vi "Variant to JSON.vi"(7 "Treatment of Infinity/NaN":T1, 8 "error in (no error)":errorcluster, 10 "Variant":variant) -> (0 "error out":errorcluster, 3 "JSON Value out":refnum<class "JSON Value.lvclass">)   [LabVIEW 2020, in "Library Commun.lvlib" / "Variant JSON.lvlib"]
doc: "Converts a LabVIEW datatype (<b>Variant</b>) into a JSON value. Clusters are converted to JSON Objects. Variants, if empty (void), are converted to null, unless they have attributes, in which case these are converted into a JSON object. \n\nTreatment of Infinity, -Infinity, and Not-a-Number values of floating-point numerics:\n<b>-- Default JSON:</b> write all as nulls.\n<b>-- Extended:</b> use JSON strings for Infinities (\"Infinity\", \"-Infinity\"); NaN still null.\n<b>-- LabVIEW extentions</b> (compatable with the LabVIEW JSON primatives): Infinity, -Infinity, NaN (not in quotes)\n\nNote that the LabVIEW extentions are not valid JSON. The Extended option <b>is</b> valid JSON, but not all JSON parsers will process strings as numeric values.\n\nMore information on http://lavag.org/topic/16217-cr-json-labview"
uses:
  Variant JSON.lvlib
  JSON Value/JSON Value.lvclass
  JSON Scalar/Infinity&NaN.ctl
  <vilib>/Utility/VariantDataType/Type.ctl
  JSON Object/JSON Object.lvclass
  C:/Users/ngarcin/OneDrive - Altyor/Standard TB/Class/JSON API/JSON Value/JSON Value.lvclass
  JSON Array/JSON Array.lvclass
  JSON Array/JSON Array.lvclass/JSON Array.ctl
  JSON Value/Set from JSON string.vi
  JSON Scalar/JSON Scalar.lvclass
  JSON Scalar/Set Null.vi
  JSON Scalar/Set I32.vi
  JSON Scalar/Set I64.vi
  JSON Scalar/Set U32.vi
  JSON Scalar/Set U64.vi
  JSON Scalar/Set SGL.vi
  JSON Scalar/Set EXT.vi
  JSON Scalar/Set Boolean.vi
  JSON Scalar/Set Path.vi
  JSON Scalar/Set Timestamp.vi
  Get Polymorphic/JSON GetSet.lvlib
  <vilib>/Utility/VariantDataType/VariantType.lvlib
  <userlib>/_OpenG.lib/lvdata/lvdata.llb/openg_variant.lvlib
  support/JSON support.lvlib
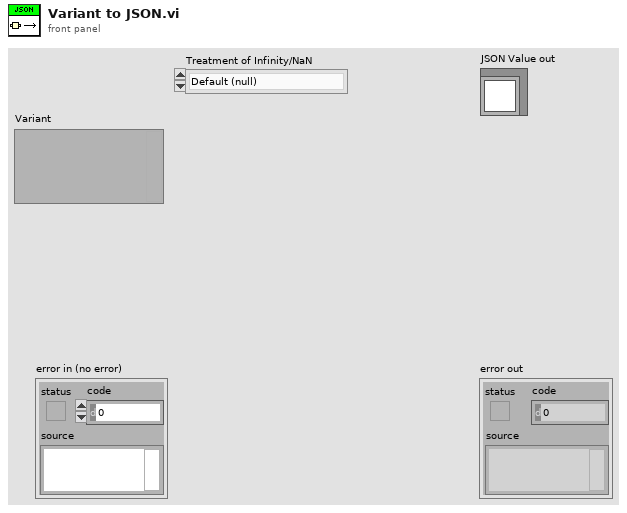
[diagram p1: front panel]
types:
  T1 = typedef "Library Commun.lvlib/JSON support.lvlib/Infinity&NaN.ctl" = enum16{"Default (null)", "Extended", "LabVIEW extensions"}
  T2 = typedef "VariantType.lvlib/Type.ctl" = enum8{"Invalid Type", "Void", "I8", "I16", "I32", "I64", "U8", "U16", "U32", "U64", "Single Float", "Double Float", "Extended Float", "Single Complex", "Double Complex", "Extended Complex", "Enum U8", "Enum U16", "Enum U32", "Enum U64", "Single Float With Unit", "Double Float With Unit", "Extended Float With Unit", "Single Complex with Unit", "Double Complex with Unit", "Extended Complex with Unit", "Boolean", "String", "Path", "Picture", "Tag", "Array", "Cluster", "Variant", "LV Variant", "Waveform", "Timestamp", "Digital Waveform", "Digital Data", "ExpressData", "Refnum", "External Data", "VI", "Poly VI", "LabVIEW Class Instance", "Fixed Point"}
  T3 = typedef "VariantType.lvlib/RefnumType.ctl" = enum16{"NotARefnum", "UnknownRefnum", "Generic", "Datalog", "ByteStream", "Device", "Occurence", "TCPNetConnection", "Auto", "Menu", "Imaq", "Hardware", "DataSocket", "Visa", "IVI", "UDPNetConnection", "Notifier", "Queue", "Irda", "EventReg", "DotNet", "UserEvent", "Callback", "UNUSED_EMPTY_POSITION", "BlueToothNetConnection", "LVObjApp", "LVObjVI", "LVObjUnknown", "GenericClass", "UserDefinedRefnumTag", "DataValue", "RT FIFO", "TDMS File"}
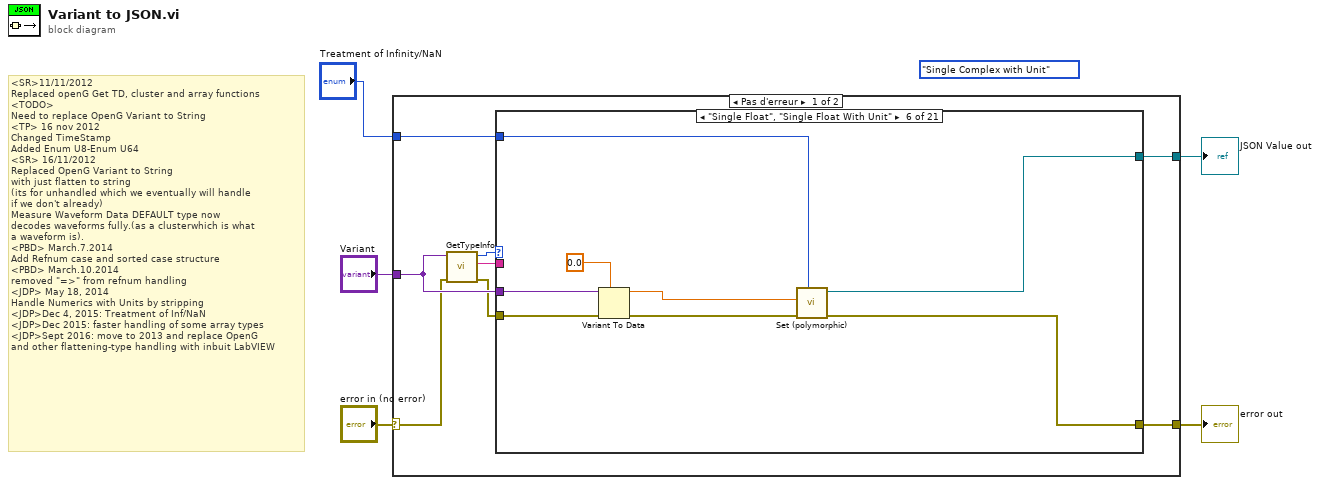
[diagram p0: block diagram]
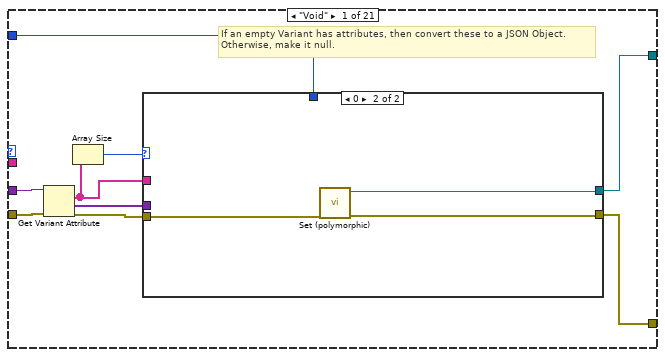
[diagram p2: hidden frame]
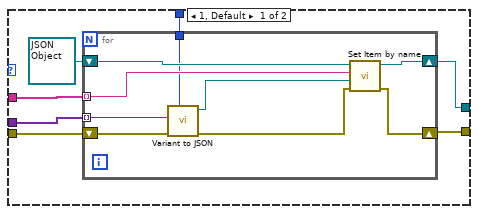
[diagram p3: hidden frame]
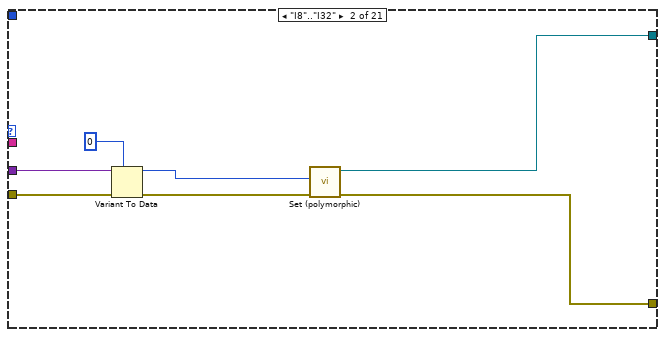
[diagram p4: hidden frame]
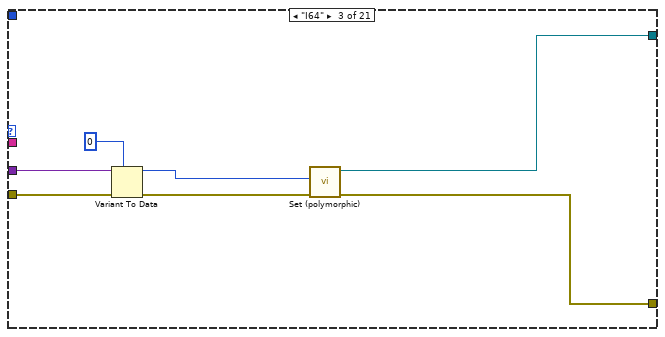
[diagram p5: hidden frame]
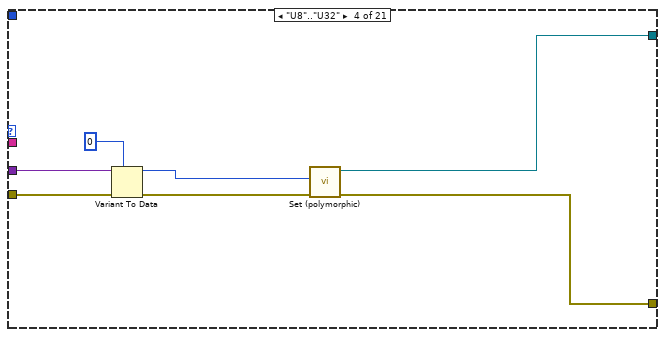
[diagram p6: hidden frame]
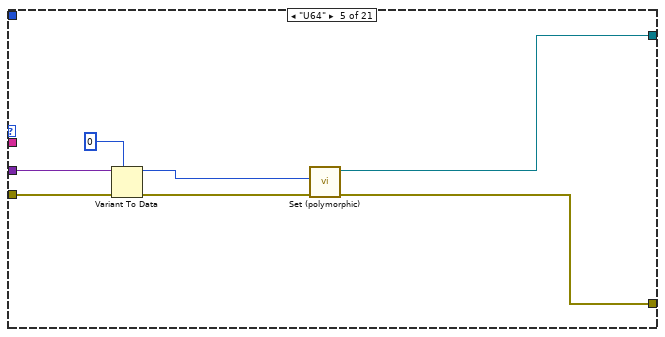
[diagram p7: hidden frame]
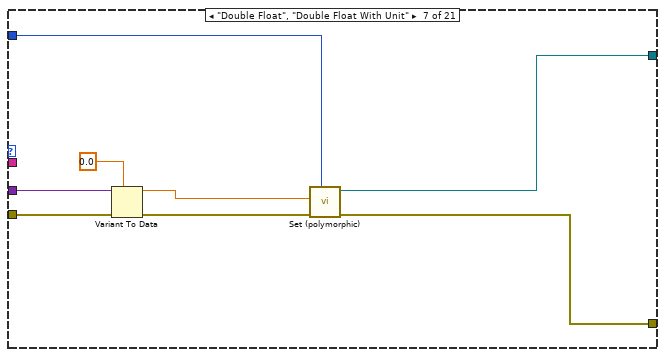
[diagram p8: hidden frame]
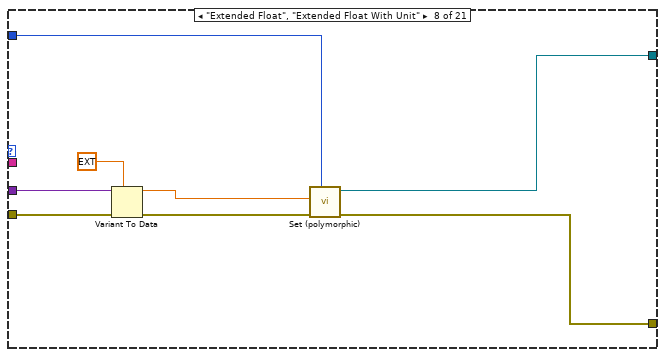
[diagram p9: hidden frame]
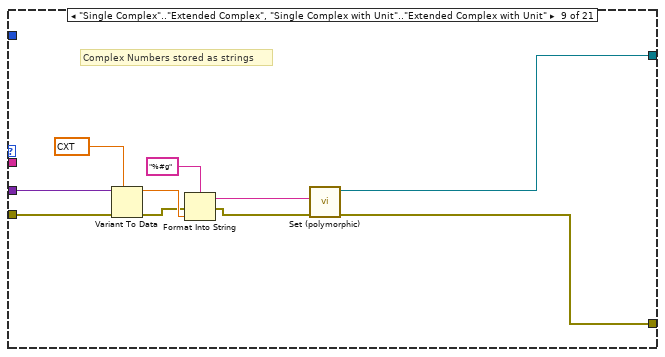
[diagram p10: hidden frame]
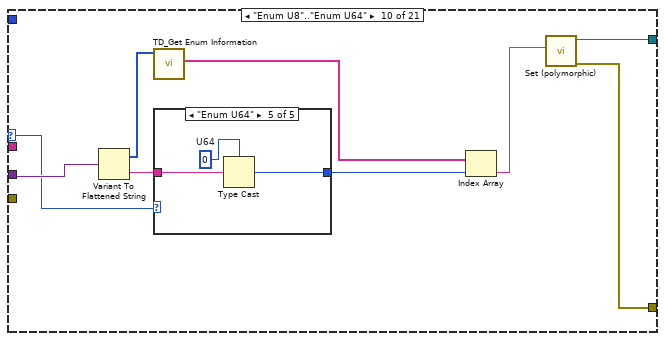
[diagram p11: hidden frame]
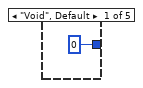
[diagram p12: hidden frame]
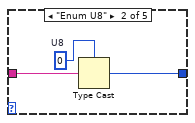
[diagram p13: hidden frame]
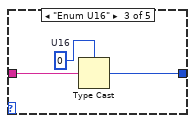
[diagram p14: hidden frame]
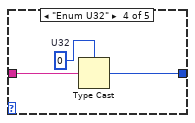
[diagram p15: hidden frame]
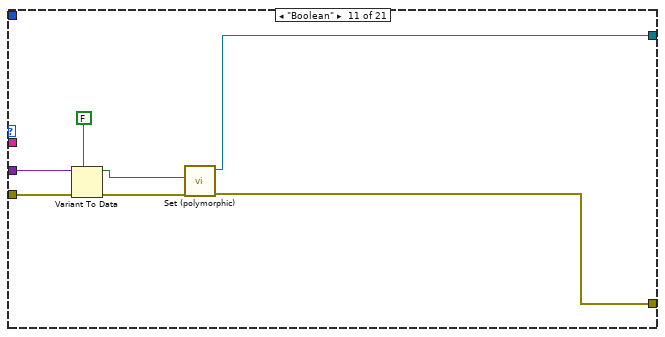
[diagram p16: hidden frame]
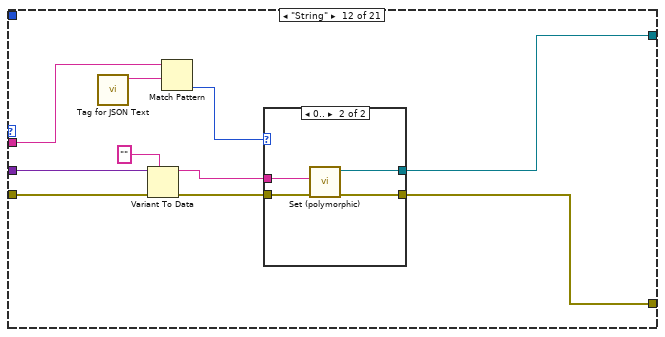
[diagram p17: hidden frame]
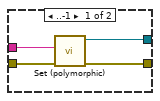
[diagram p18: hidden frame]
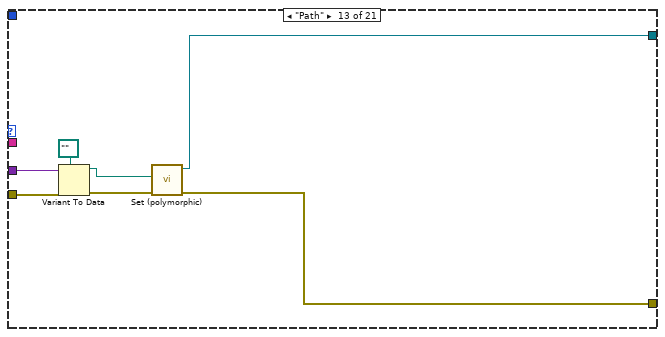
[diagram p19: hidden frame]
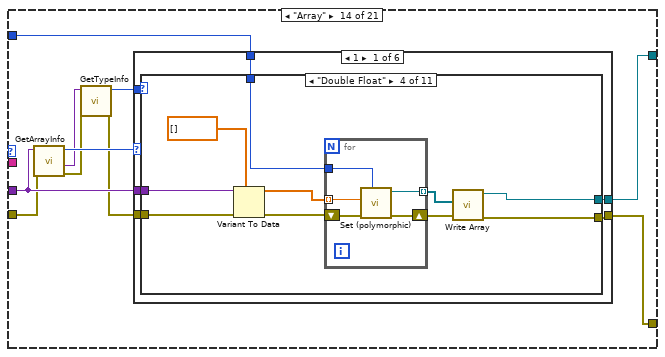
[diagram p20: hidden frame]
diagram:
  (unwired) Type."Single Complex with Unit" ("Type Enum")
  # "<SR>11/11/2012\nReplaced openG Get TD, cluster and array functions\n<TODO>\nNeed to replace OpenG Variant to String\n<TP> 16 nov 2012\nChanged TimeStamp\nAdded Enum U8-Enum U64\n<SR> 16/11/2012\nReplaced OpenG Variant to String\nwith just flatten to string \n(its for unhandled which we eventually will handle\nif we don't already)\nMeasure Waveform Data DEFAULT type now \ndecodes waveforms fully.(as a clusterwhich is what\na waveform is).\n<PBD> March.7.2014\nAdd Refnum case and sorted case structure\n<PBD> March.10.2014\nremoved \"=>\" from refnum handling\n<JDP> May 18, 2014\nHandle Numerics with Units by stripping\n<JDP>Dec 4, 2015: Treatment of Inf/NaN\n<JDP>Dec 2015: faster handling of some array types\n<JDP>Sept 2016: move to 2013 and replace OpenG\nand other flattening-type handling with inbuit LabVIEW"
  n1 = case shown="Pas d'erreur" "error in (no error)" {
    selector: "error in (no error)" -> [w10 w664]
    tunnel: [w12 w664] -> w4
    tunnel: [w13 _] -> w3
    tunnel: "Variant" -> [w11 _]
    tunnel: "Treatment of Infinity/NaN" -> [w6 _]
    frame No Error {
      n2 = call <vilib>:"GetTypeInfo.vi"("error in (no error)"=w10, "Variant"=w11) -> ("error out"=w9:errorcluster, "Name"=w7:string, "Type Enum"=w8:T2)  [unwired: 5 in, 2 out]
      n3 = case shown="\"Single Float\", \"Single Float With Unit\"" w8 {
        selector: w8 -> [_ _ _ _ _ _ _ _ _ w105 _ _ _ _ _ _ _ _ _ _ _]
        tunnel: w11 -> [w20 w48 w55 w62 w69 w77 w85 w93 w103 w106 w132 w142 w157 w164 w557 w594 w605 w612 w618 w648 w660]
        tunnel: [w22 w45 w52 w59 w66 w74 w82 w90 w102 w112 w129 w139 w153 w166 w559 w599 w607 w614 w616 w642 w663] -> w13
        tunnel: [w21 w43 w50 w57 w64 w72 w80 w88 w101 w111 w127 w137 w152 w167 w558 w598 w606 w613 w615 w641 w662] -> w12
        tunnel: w9 -> [w15 w42 w49 w56 w63 w71 w79 w87 w100 _ w126 w136 w155 w163 w555 w593 w604 w608 w617 w647 w661]
        tunnel: w7 -> [_ _ _ _ _ _ _ _ _ _ _ w134 _ _ _ _ _ _ _ _ _]
        tunnel: w6 -> [w14 _ _ _ _ w70 w78 w86 _ _ _ _ _ w165 w554 w592 w603 _ _ _ _]
        frame "Void" {
          # "If an empty Variant has attributes, then convert these to a JSON Object.\nOtherwise, make it null."
          n4 = Get Variant Attribute(Variant=w20, error in=w15) -> (names=w18:string[], values=w17:variant[], error out=w16:errorcluster)  [unwired: 2 in, 1 out]
          n5 = Array Size(array=w18) -> (size(s)=w19:i32)
          n6 = case shown="0" w19 {
            tunnel: [w25 w40] -> w21
            tunnel: [w24 w41] -> w22
            tunnel: w18 -> [w27 _]
            tunnel: w17 -> [w29 _]
            tunnel: w16 -> [w28 w39]
            tunnel: w14 -> [w23 _]
            frame 1, Default {
              n7 = for {
                tunnel: w29 -> [w35] mode=indexing
                shift-right: [w31] -> w25
                shift-left: w28 -> [w34]
                tunnel: w27 -> [w36] mode=indexing
                shift-right: [w38] -> w24
                shift-left: refnum<class "JSON Object.lvclass"> refnum ("JSON Object out") -> [w37]
                tunnel: w23 -> [w30]
                n8 = call "Variant to JSON.vi"("Treatment of Infinity/NaN"=w30, "error in (no error)"=w34, "Variant"=w35) -> ("error out"=w32:errorcluster, "JSON Value out"=w33:refnum<class "JSON Value.lvclass">)  [unwired: 7 in]
                n9 = call-dynamic "Set Item by name.vi"("error in (no error)"=w32, "Value"=w33, "name"=w36, "JSON Object in"=w37) -> ("error out"=w31:errorcluster, "JSON Object out"=w38:refnum<class "JSON Object.lvclass">)  [unwired: 5 in, 1 out]
              }
            }
            frame 0 {
              n10 = call-poly "Set (polymorphic).vi"("error in (no error)"=w39) -> ("error out"=w40:errorcluster, "JSON Scalar out"=w41:refnum<class "JSON Scalar.lvclass">)  [unwired: 9 in]
            }
          }
        }
        frame "I8".."I32" {
          n11 = Variant To Data(error in=w42, type=0, Variant=w48) -> (data=w46:i32, error out=w44:errorcluster)
          n12 = call-poly "Set (polymorphic).vi"("error in (no error)"=w44, "Numeric"=w46) -> ("error out"=w43:errorcluster, "JSON Scalar out"=w45:refnum<class "JSON Scalar.lvclass">)  [unwired: 8 in]
        }
        frame "I64" {
          n13 = Variant To Data(error in=w49, type=i64 0, Variant=w55) -> (data=w53:i64, error out=w51:errorcluster)
          n14 = call-poly "Set (polymorphic).vi"("error in (no error)"=w51, "Numeric"=w53) -> ("error out"=w50:errorcluster, "JSON Scalar out"=w52:refnum<class "JSON Scalar.lvclass">)  [unwired: 8 in]
        }
        frame "U8".."U32" {
          n15 = Variant To Data(error in=w56, type=u32 0, Variant=w62) -> (data=w60:u32, error out=w58:errorcluster)
          n16 = call-poly "Set (polymorphic).vi"("error in (no error)"=w58, "Numeric"=w60) -> ("error out"=w57:errorcluster, "JSON Scalar out"=w59:refnum<class "JSON Scalar.lvclass">)  [unwired: 8 in]
        }
        frame "U64" {
          n17 = Variant To Data(error in=w63, type=u64 0, Variant=w69) -> (data=w67:u64, error out=w65:errorcluster)
          n18 = call-poly "Set (polymorphic).vi"("error in (no error)"=w65, "Numeric"=w67) -> ("error out"=w64:errorcluster, "JSON Scalar out"=w66:refnum<class "JSON Scalar.lvclass">)  [unwired: 8 in]
        }
        frame "Single Float", "Single Float With Unit" {
          n19 = Variant To Data(error in=w71, type=sgl 0.0, Variant=w77) -> (data=w75:sgl, error out=w73:errorcluster)
          n20 = call-poly "Set (polymorphic).vi"("Treatment of Infinity/NaN"=w70, "error in (no error)"=w73, "Numeric"=w75) -> ("error out"=w72:errorcluster, "JSON Scalar out"=w74:refnum<class "JSON Scalar.lvclass">)  [unwired: 7 in]
        }
        frame "Double Float", "Double Float With Unit" {
          n21 = Variant To Data(error in=w79, type=0.0, Variant=w85) -> (data=w83:dbl, error out=w81:errorcluster)
          n22 = call-poly "Set (polymorphic).vi"("Treatment of Infinity/NaN"=w78, "error in (no error)"=w81, "Numeric"=w83) -> ("error out"=w80:errorcluster, "JSON Scalar out"=w82:refnum<class "JSON Scalar.lvclass">)  [unwired: 7 in]
        }
        frame "Extended Float", "Extended Float With Unit" {
          n23 = Variant To Data(error in=w87, type=ext 0.0, Variant=w93) -> (data=w91:ext, error out=w89:errorcluster)
          n24 = call-poly "Set (polymorphic).vi"("Treatment of Infinity/NaN"=w86, "error in (no error)"=w89, "Numeric"=w91) -> ("error out"=w88:errorcluster, "JSON Scalar out"=w90:refnum<class "JSON Scalar.lvclass">)  [unwired: 7 in]
        }
        frame "Single Complex".."Extended Complex", "Single Complex with Unit".."Extended Complex with Unit" {
          # "Complex Numbers stored as strings"
          n25 = Variant To Data(error in=w100, type=cxt 0.0+0.0i, Variant=w103) -> (data=w98:cxt, error out=w96:errorcluster)
          n26 = Format Into String(format string="%#g", error in=w96, w98) -> (resulting string=w97:string, error out=w95:errorcluster)  [unwired: 1 in]
          n27 = call-poly "Set (polymorphic).vi"("error in (no error)"=w95, "String"=w97) -> ("error out"=w101:errorcluster, "JSON Scalar out"=w102:refnum<class "JSON Scalar.lvclass">)  [unwired: 8 in]
        }
        frame "Enum U8".."Enum U64" {
          n28 = Variant To Flattened String(Variant=w106) -> (data string=w109:string, 1:w110:i16[])
          n29 = call <vilib>:"TD_Get Enum Information.vi"("Type descriptor"=w110) -> ("Value Names"=w108:string[])  [unwired: 9 in, 1 out]
          n30 = case shown="\"Enum U64\"" w105 {
            tunnel: w109 -> [_ w116 w119 w122 w125]
            tunnel: [u64 0 ("U8") w114 w117 w120 w123] -> w107
            frame "Void", Default {
            }
            frame "Enum U8" {
              w115 = u8 0  # U8
              n31 = Type Cast(type=w115, x=w116) -> (*(type *) &x=w114:u8)
            }
            frame "Enum U16" {
              w118 = u16 0  # U16
              n32 = Type Cast(type=w118, x=w119) -> (*(type *) &x=w117:u16)
            }
            frame "Enum U32" {
              w121 = u32 0  # U32
              n33 = Type Cast(type=w121, x=w122) -> (*(type *) &x=w120:u32)
            }
            frame "Enum U64" {
              w124 = u64 0  # U64
              n34 = Type Cast(type=w124, x=w125) -> (*(type *) &x=w123:u64)
            }
          }
          n35 = Index Array(array=w108, index=w107) -> (element=w104:string)
          n36 = call-poly "Set (polymorphic).vi"("String"=w104) -> ("error out"=w111:errorcluster, "JSON Scalar out"=w112:refnum<class "JSON Scalar.lvclass">)  [unwired: 9 in]
        }
        frame "Boolean" {
          n37 = Variant To Data(error in=w126, type=FALSE, Variant=w132) -> (data=w130:bool, error out=w128:errorcluster)
          n38 = call-poly "Set (polymorphic).vi"("error in (no error)"=w128, "Boolean"=w130) -> ("error out"=w127:errorcluster, "JSON Scalar out"=w129:refnum<class "JSON Scalar.lvclass">)  [unwired: 8 in]
        }
        frame "String" {
          n39 = call "Tag for JSON Text.vi"() -> ("Tag for JSON text"=w135:string)  [unwired: 11 in]
          n40 = Variant To Data(error in=w136, type="", Variant=w142) -> (data=w140:string, error out=w138:errorcluster)
          n41 = Match Pattern(string=w134, regular expression=w135) -> (offset past match=w133:i32)  [unwired: 1 in, 3 out]
          n42 = case shown="0.." w133 {
            tunnel: w140 -> [w146 w150]
            tunnel: [w145 w149] -> w139
            tunnel: w138 -> [w144 w148]
            tunnel: [w143 w147] -> w137
            frame ..-1 {
              n43 = call-poly "Set (polymorphic).vi"("error in (no error)"=w144, "String"=w146) -> ("error out"=w143:errorcluster, "JSON Scalar out"=w145:refnum<class "JSON Scalar.lvclass">)  [unwired: 8 in]
            }
            frame 0.. {
              n44 = call-poly "Set (polymorphic).vi"("error in (no error)"=w148, "JSON stream"=w150) -> ("error out"=w147:errorcluster, "JSON Value out"=w149:refnum<class "JSON Value.lvclass">)  [unwired: 7 in, 1 out]
            }
          }
        }
        frame "Path" {
          n45 = Variant To Data(error in=w155, type=path "", Variant=w157) -> (data=w151:path, error out=w154:errorcluster)
          n46 = call-poly "Set (polymorphic).vi"("error in (no error)"=w154, "Path"=w151) -> ("error out"=w152:errorcluster, "JSON Scalar out"=w153:refnum<class "JSON Scalar.lvclass">)  [unwired: 8 in]
        }
        frame "Array" {
          n47 = call <vilib>:"GetArrayInfo.vi"("error in (no error)"=w163, "Variant"=w164) -> ("error out"=w161:errorcluster, "ArrayElement"=w160:variant, "NDims"=w162:i32)  [unwired: 6 in, 1 out]
          n48 = call <vilib>:"GetTypeInfo.vi"("error in (no error)"=w161, "Variant"=w160) -> ("error out"=w159:errorcluster, "Type Enum"=w158:T2)  [unwired: 5 in, 3 out]
          n49 = case shown="1" w162 {
            tunnel: [w172 w332 w506 w521 w536 w549] -> w167
            tunnel: [w171 w331 w505 w520 w535 w548] -> w166
            tunnel: w165 -> [w169 w329 w503 w518 w533 w547]
            tunnel: w164 -> [w173 w333 w507 w522 w537 _]
            tunnel: w159 -> [w170 w330 w504 w519 w534 w546]
            tunnel: w158 -> [w168 w328 _ _ _ _]
            frame 1 {
              n50 = case shown="\"Double Float\"" w168 {
                tunnel: w173 -> [w184 w198 w212 w227 w242 w256 w269 w282 w295 w308 w322]
                tunnel: [w178 w192 w206 w221 w236 w250 w263 w276 w289 w302 w316] -> w172
                tunnel: [w177 w191 w205 w220 w235 w249 w262 w275 w288 w301 w315] -> w171
                tunnel: w170 -> [w175 w190 w204 w219 w234 w248 w261 w274 w287 w300 w314]
                tunnel: w169 -> [w174 _ w203 w218 w233 _ _ _ _ _ w313]
                frame Default {
                  n51 = Variant To Data(error in=w175, type=variant[] [], Variant=w184) -> (data=w182:variant[], error out=w181:errorcluster)
                  n52 = for {
                    tunnel: w182 -> [w189] mode=indexing
                    shift-right: [w187] -> w179
                    shift-left: w181 -> [w188]
                    tunnel: [w186] -> w180 mode=indexing
                    tunnel: w174 -> [w185]
                    n53 = call "Variant to JSON.vi"("Treatment of Infinity/NaN"=w185, "error in (no error)"=w188, "Variant"=w189) -> ("error out"=w187:errorcluster, "JSON Value out"=w186:refnum<class "JSON Value.lvclass">)  [unwired: 7 in]
                  }
                  n54 = call "Write Array.vi"("error in (no error)"=w179, "Array"=w180, "JSON Array in"=refnum<class "JSON Array.lvclass"> refnum) -> ("error out"=w178:errorcluster, "JSON Array out"=w177:refnum<class "JSON Array.lvclass">)  [unwired: 7 in]
                }
                frame "String" {
                  n55 = Variant To Data(error in=w190, type=string[] [], Variant=w198) -> (data=w196:string[], error out=w195:errorcluster)
                  n56 = for {
                    tunnel: w196 -> [w199] mode=indexing
                    shift-right: [w201] -> w193
                    shift-left: w195 -> [w202]
                    tunnel: [w200] -> w194 mode=indexing
                    n57 = call "Set String.vi"("error in (no error)"=w202, "String"=w199) -> ("error out"=w201:errorcluster, "JSON Scalar out"=w200:refnum<class "JSON Scalar.lvclass">)  [unwired: 8 in]
                  }
                  n58 = call "Write Array.vi"("error in (no error)"=w193, "Array"=w194) -> ("error out"=w192:errorcluster, "JSON Array out"=w191:refnum<class "JSON Array.lvclass">)  [unwired: 8 in]
                }
                frame "Single Float" {
                  n59 = Variant To Data(error in=w204, type=sgl[] [], Variant=w212) -> (data=w210:sgl[], error out=w209:errorcluster)
                  n60 = for {
                    tunnel: w210 -> [w213] mode=indexing
                    shift-right: [w216] -> w207
                    shift-left: w209 -> [w217]
                    tunnel: [w215] -> w208 mode=indexing
                    tunnel: w203 -> [w214]
                    n61 = call "Set DBL.vi"("Treatment of Infinity/NaN"=w214, "error in (no error)"=w217, "Numeric"=w213) -> ("error out"=w216:errorcluster, "JSON Scalar out"=w215:refnum<class "JSON Scalar.lvclass">)  [unwired: 7 in]
                  }
                  n62 = call "Write Array.vi"("error in (no error)"=w207, "Array"=w208) -> ("error out"=w206:errorcluster, "JSON Array out"=w205:refnum<class "JSON Array.lvclass">)  [unwired: 8 in]
                }
                frame "Double Float" {
                  n63 = Variant To Data(error in=w219, type=dbl[] [], Variant=w227) -> (data=w225:dbl[], error out=w224:errorcluster)
                  n64 = for {
                    tunnel: w225 -> [w228] mode=indexing
                    shift-right: [w231] -> w222
                    shift-left: w224 -> [w232]
                    tunnel: [w230] -> w223 mode=indexing
                    tunnel: w218 -> [w229]
                    n65 = call-poly "Set (polymorphic).vi"("Treatment of Infinity/NaN"=w229, "error in (no error)"=w232, "Numeric"=w228) -> ("error out"=w231:errorcluster, "JSON Scalar out"=w230:refnum<class "JSON Scalar.lvclass">)  [unwired: 7 in]
                  }
                  n66 = call "Write Array.vi"("error in (no error)"=w222, "Array"=w223) -> ("error out"=w221:errorcluster, "JSON Array out"=w220:refnum<class "JSON Array.lvclass">)  [unwired: 8 in]
                }
                frame "Extended Float" {
                  n67 = Variant To Data(error in=w234, type=ext[] [], Variant=w242) -> (data=w240:ext[], error out=w239:errorcluster)
                  n68 = for {
                    tunnel: w240 -> [w243] mode=indexing
                    shift-right: [w246] -> w237
                    shift-left: w239 -> [w247]
                    tunnel: [w245] -> w238 mode=indexing
                    tunnel: w233 -> [w244]
                    n69 = call-poly "Set (polymorphic).vi"("Treatment of Infinity/NaN"=w244, "error in (no error)"=w247, "Numeric"=w243) -> ("error out"=w246:errorcluster, "JSON Scalar out"=w245:refnum<class "JSON Scalar.lvclass">)  [unwired: 7 in]
                  }
                  n70 = call "Write Array.vi"("error in (no error)"=w237, "Array"=w238) -> ("error out"=w236:errorcluster, "JSON Array out"=w235:refnum<class "JSON Array.lvclass">)  [unwired: 8 in]
                }
                frame "I8".."I32" {
                  n71 = Variant To Data(error in=w248, type=i32[] [], Variant=w256) -> (data=w254:i32[], error out=w253:errorcluster)
                  n72 = for {
                    tunnel: w254 -> [w257] mode=indexing
                    shift-right: [w259] -> w251
                    shift-left: w253 -> [w260]
                    tunnel: [w258] -> w252 mode=indexing
                    n73 = call-poly "Set (polymorphic).vi"("error in (no error)"=w260, "Numeric"=w257) -> ("error out"=w259:errorcluster, "JSON Scalar out"=w258:refnum<class "JSON Scalar.lvclass">)  [unwired: 8 in]
                  }
                  n74 = call "Write Array.vi"("error in (no error)"=w251, "Array"=w252) -> ("error out"=w250:errorcluster, "JSON Array out"=w249:refnum<class "JSON Array.lvclass">)  [unwired: 8 in]
                }
                frame "I64" {
                  n75 = Variant To Data(error in=w261, type=i64[] [], Variant=w269) -> (data=w267:i64[], error out=w266:errorcluster)
                  n76 = for {
                    tunnel: w267 -> [w270] mode=indexing
                    shift-right: [w272] -> w264
                    shift-left: w266 -> [w273]
                    tunnel: [w271] -> w265 mode=indexing
                    n77 = call-poly "Set (polymorphic).vi"("error in (no error)"=w273, "Numeric"=w270) -> ("error out"=w272:errorcluster, "JSON Scalar out"=w271:refnum<class "JSON Scalar.lvclass">)  [unwired: 8 in]
                  }
                  n78 = call "Write Array.vi"("error in (no error)"=w264, "Array"=w265) -> ("error out"=w263:errorcluster, "JSON Array out"=w262:refnum<class "JSON Array.lvclass">)  [unwired: 8 in]
                }
                frame "U8".."U32" {
                  n79 = Variant To Data(error in=w274, type=u32[] [], Variant=w282) -> (data=w280:u32[], error out=w279:errorcluster)
                  n80 = for {
                    tunnel: w280 -> [w283] mode=indexing
                    shift-right: [w285] -> w277
                    shift-left: w279 -> [w286]
                    tunnel: [w284] -> w278 mode=indexing
                    n81 = call-poly "Set (polymorphic).vi"("error in (no error)"=w286, "Numeric"=w283) -> ("error out"=w285:errorcluster, "JSON Scalar out"=w284:refnum<class "JSON Scalar.lvclass">)  [unwired: 8 in]
                  }
                  n82 = call "Write Array.vi"("error in (no error)"=w277, "Array"=w278) -> ("error out"=w276:errorcluster, "JSON Array out"=w275:refnum<class "JSON Array.lvclass">)  [unwired: 8 in]
                }
                frame "U64" {
                  n83 = Variant To Data(error in=w287, type=u64[] [], Variant=w295) -> (data=w293:u64[], error out=w292:errorcluster)
                  n84 = for {
                    tunnel: w293 -> [w296] mode=indexing
                    shift-right: [w298] -> w290
                    shift-left: w292 -> [w299]
                    tunnel: [w297] -> w291 mode=indexing
                    n85 = call-poly "Set (polymorphic).vi"("error in (no error)"=w299, "Numeric"=w296) -> ("error out"=w298:errorcluster, "JSON Scalar out"=w297:refnum<class "JSON Scalar.lvclass">)  [unwired: 8 in]
                  }
                  n86 = call "Write Array.vi"("error in (no error)"=w290, "Array"=w291) -> ("error out"=w289:errorcluster, "JSON Array out"=w288:refnum<class "JSON Array.lvclass">)  [unwired: 8 in]
                }
                frame "Timestamp" {
                  n87 = Variant To Data(error in=w300, type=timestamp[] [], Variant=w308) -> (data=w306:timestamp[], error out=w305:errorcluster)
                  n88 = for {
                    tunnel: w306 -> [w309] mode=indexing
                    shift-right: [w311] -> w303
                    shift-left: w305 -> [w312]
                    tunnel: [w310] -> w304 mode=indexing
                    n89 = call-poly "Set (polymorphic).vi"("error in (no error)"=w312, "Time Stamp"=w309) -> ("error out"=w311:errorcluster, "JSON Scalar out"=w310:refnum<class "JSON Scalar.lvclass">)  [unwired: 8 in]
                  }
                  n90 = call "Write Array.vi"("error in (no error)"=w303, "Array"=w304) -> ("error out"=w302:errorcluster, "JSON Array out"=w301:refnum<class "JSON Array.lvclass">)  [unwired: 8 in]
                }
                frame "Waveform" {
                  n91 = Variant To Data(error in=w314, type=waveform(dbl)[] [], Variant=w322) -> (data=w320:waveform(dbl)[], error out=w319:errorcluster)
                  n92 = for {
                    tunnel: w320 -> [w324] mode=indexing
                    shift-right: [w326] -> w317
                    shift-left: w319 -> [w327]
                    tunnel: [w325] -> w318 mode=indexing
                    tunnel: w313 -> [w323]
                    n93 = call-poly "Set (polymorphic).vi"("Treatment of Infinity/NaN"=w323, "error in (no error)"=w327, "waveform"=w324) -> ("error out"=w326:errorcluster, "JSON Object out"=w325:refnum<class "JSON Object.lvclass">)  [unwired: 7 in]
                  }
                  n94 = call "Write Array.vi"("error in (no error)"=w317, "Array"=w318) -> ("error out"=w316:errorcluster, "JSON Array out"=w315:refnum<class "JSON Array.lvclass">)  [unwired: 8 in]
                }
              }
            }
            frame 2 {
              n95 = case shown="\"Extended Float\"" w328 {
                tunnel: w333 -> [w343 w365 w387 w409 w430 w449 w468 w487]
                tunnel: [w336 w358 w380 w402 w424 w443 w462 w481] -> w332
                tunnel: [w335 w357 w379 w401 w423 w442 w461 w480] -> w331
                tunnel: w330 -> [w340 w362 w384 w406 w427 w446 w465 w484]
                tunnel: w329 -> [w339 w361 w383 w405 _ _ _ _]
                frame Default {
                  n96 = Variant To Data(error in=w340, type=variant[][] [], Variant=w343) -> (data=w341:variant[][], error out=w334:errorcluster)
                  n97 = for {
                    tunnel: w341 -> [w350] mode=indexing
                    tunnel: [w346] -> w338 mode=indexing
                    tunnel: w339 -> [w345]
                    shift-right: [w347] -> w337
                    shift-left: w334 -> [w344]
                    n98 = for {
                      tunnel: w350 -> [w355] mode=indexing
                      shift-right: [w353] -> w348
                      shift-left: w344 -> [w354]
                      tunnel: [w352] -> w349 mode=indexing
                      tunnel: w345 -> [w351]
                      n99 = call "Variant to JSON.vi"("Treatment of Infinity/NaN"=w351, "error in (no error)"=w354, "Variant"=w355) -> ("error out"=w353:errorcluster, "JSON Value out"=w352:refnum<class "JSON Value.lvclass">)  [unwired: 7 in]
                    }
                    n100 = call "Write Array.vi"("error in (no error)"=w348, "Array"=w349) -> ("error out"=w347:errorcluster, "JSON Array out"=w346:refnum<class "JSON Array.lvclass">)  [unwired: 8 in]
                  }
                  n101 = call "Write Array.vi"("error in (no error)"=w337, "Array"=w338) -> ("error out"=w336:errorcluster, "JSON Array out"=w335:refnum<class "JSON Array.lvclass">)  [unwired: 8 in]
                }
                frame "Double Float" {
                  n102 = Variant To Data(error in=w362, type=dbl[][] [], Variant=w365) -> (data=w363:dbl[][], error out=w356:errorcluster)
                  n103 = for {
                    tunnel: w363 -> [w372] mode=indexing
                    tunnel: [w368] -> w360 mode=indexing
                    tunnel: w361 -> [w367]
                    shift-right: [w369] -> w359
                    shift-left: w356 -> [w366]
                    n104 = for {
                      tunnel: w372 -> [w373] mode=indexing
                      shift-right: [w376] -> w370
                      shift-left: w366 -> [w377]
                      tunnel: [w375] -> w371 mode=indexing
                      tunnel: w367 -> [w374]
                      n105 = call "Set DBL.vi"("Treatment of Infinity/NaN"=w374, "error in (no error)"=w377, "Numeric"=w373) -> ("error out"=w376:errorcluster, "JSON Scalar out"=w375:refnum<class "JSON Scalar.lvclass">)  [unwired: 7 in]
                    }
                    n106 = call "Write Array.vi"("error in (no error)"=w370, "Array"=w371) -> ("error out"=w369:errorcluster, "JSON Array out"=w368:refnum<class "JSON Array.lvclass">)  [unwired: 8 in]
                  }
                  n107 = call "Write Array.vi"("error in (no error)"=w359, "Array"=w360) -> ("error out"=w358:errorcluster, "JSON Array out"=w357:refnum<class "JSON Array.lvclass">)  [unwired: 8 in]
                }
                frame "Single Float" {
                  n108 = Variant To Data(error in=w384, type=sgl[][] [], Variant=w387) -> (data=w385:sgl[][], error out=w378:errorcluster)
                  n109 = for {
                    tunnel: w385 -> [w394] mode=indexing
                    tunnel: [w390] -> w382 mode=indexing
                    tunnel: w383 -> [w389]
                    shift-right: [w391] -> w381
                    shift-left: w378 -> [w388]
                    n110 = for {
                      tunnel: w394 -> [w395] mode=indexing
                      shift-right: [w398] -> w392
                      shift-left: w388 -> [w399]
                      tunnel: [w397] -> w393 mode=indexing
                      tunnel: w389 -> [w396]
                      n111 = call-poly "Set (polymorphic).vi"("Treatment of Infinity/NaN"=w396, "error in (no error)"=w399, "Numeric"=w395) -> ("error out"=w398:errorcluster, "JSON Scalar out"=w397:refnum<class "JSON Scalar.lvclass">)  [unwired: 7 in]
                    }
                    n112 = call "Write Array.vi"("error in (no error)"=w392, "Array"=w393) -> ("error out"=w391:errorcluster, "JSON Array out"=w390:refnum<class "JSON Array.lvclass">)  [unwired: 8 in]
                  }
                  n113 = call "Write Array.vi"("error in (no error)"=w381, "Array"=w382) -> ("error out"=w380:errorcluster, "JSON Array out"=w379:refnum<class "JSON Array.lvclass">)  [unwired: 8 in]
                }
                frame "Extended Float" {
                  n114 = Variant To Data(error in=w406, type=ext[][] [], Variant=w409) -> (data=w407:ext[][], error out=w400:errorcluster)
                  n115 = for {
                    tunnel: w407 -> [w416] mode=indexing
                    tunnel: [w412] -> w404 mode=indexing
                    tunnel: w405 -> [w411]
                    shift-right: [w413] -> w403
                    shift-left: w400 -> [w410]
                    n116 = for {
                      tunnel: w416 -> [w417] mode=indexing
                      shift-right: [w420] -> w414
                      shift-left: w410 -> [w421]
                      tunnel: [w419] -> w415 mode=indexing
                      tunnel: w411 -> [w418]
                      n117 = call-poly "Set (polymorphic).vi"("Treatment of Infinity/NaN"=w418, "error in (no error)"=w421, "Numeric"=w417) -> ("error out"=w420:errorcluster, "JSON Scalar out"=w419:refnum<class "JSON Scalar.lvclass">)  [unwired: 7 in]
                    }
                    n118 = call "Write Array.vi"("error in (no error)"=w414, "Array"=w415) -> ("error out"=w413:errorcluster, "JSON Array out"=w412:refnum<class "JSON Array.lvclass">)  [unwired: 8 in]
                  }
                  n119 = call "Write Array.vi"("error in (no error)"=w403, "Array"=w404) -> ("error out"=w402:errorcluster, "JSON Array out"=w401:refnum<class "JSON Array.lvclass">)  [unwired: 8 in]
                }
                frame "I8".."I32" {
                  n120 = Variant To Data(error in=w427, type=i32[][] [], Variant=w430) -> (data=w428:i32[][], error out=w422:errorcluster)
                  n121 = for {
                    tunnel: w428 -> [w436] mode=indexing
                    tunnel: [w432] -> w426 mode=indexing
                    shift-right: [w433] -> w425
                    shift-left: w422 -> [w431]
                    n122 = for {
                      tunnel: w436 -> [w437] mode=indexing
                      shift-right: [w439] -> w434
                      shift-left: w431 -> [w440]
                      tunnel: [w438] -> w435 mode=indexing
                      n123 = call-poly "Set (polymorphic).vi"("error in (no error)"=w440, "Numeric"=w437) -> ("error out"=w439:errorcluster, "JSON Scalar out"=w438:refnum<class "JSON Scalar.lvclass">)  [unwired: 8 in]
                    }
                    n124 = call "Write Array.vi"("error in (no error)"=w434, "Array"=w435) -> ("error out"=w433:errorcluster, "JSON Array out"=w432:refnum<class "JSON Array.lvclass">)  [unwired: 8 in]
                  }
                  n125 = call "Write Array.vi"("error in (no error)"=w425, "Array"=w426) -> ("error out"=w424:errorcluster, "JSON Array out"=w423:refnum<class "JSON Array.lvclass">)  [unwired: 8 in]
                }
                frame "I64" {
                  n126 = Variant To Data(error in=w446, type=i64[][] [], Variant=w449) -> (data=w447:i64[][], error out=w441:errorcluster)
                  n127 = for {
                    tunnel: w447 -> [w455] mode=indexing
                    tunnel: [w451] -> w445 mode=indexing
                    shift-right: [w452] -> w444
                    shift-left: w441 -> [w450]
                    n128 = for {
                      tunnel: w455 -> [w456] mode=indexing
                      shift-right: [w458] -> w453
                      shift-left: w450 -> [w459]
                      tunnel: [w457] -> w454 mode=indexing
                      n129 = call-poly "Set (polymorphic).vi"("error in (no error)"=w459, "Numeric"=w456) -> ("error out"=w458:errorcluster, "JSON Scalar out"=w457:refnum<class "JSON Scalar.lvclass">)  [unwired: 8 in]
                    }
                    n130 = call "Write Array.vi"("error in (no error)"=w453, "Array"=w454) -> ("error out"=w452:errorcluster, "JSON Array out"=w451:refnum<class "JSON Array.lvclass">)  [unwired: 8 in]
                  }
                  n131 = call "Write Array.vi"("error in (no error)"=w444, "Array"=w445) -> ("error out"=w443:errorcluster, "JSON Array out"=w442:refnum<class "JSON Array.lvclass">)  [unwired: 8 in]
                }
                frame "U8".."U32" {
                  n132 = Variant To Data(error in=w465, type=u32[][] [], Variant=w468) -> (data=w466:u32[][], error out=w460:errorcluster)
                  n133 = for {
                    tunnel: w466 -> [w474] mode=indexing
                    tunnel: [w470] -> w464 mode=indexing
                    shift-right: [w471] -> w463
                    shift-left: w460 -> [w469]
                    n134 = for {
                      tunnel: w474 -> [w475] mode=indexing
                      shift-right: [w477] -> w472
                      shift-left: w469 -> [w478]
                      tunnel: [w476] -> w473 mode=indexing
                      n135 = call-poly "Set (polymorphic).vi"("error in (no error)"=w478, "Numeric"=w475) -> ("error out"=w477:errorcluster, "JSON Scalar out"=w476:refnum<class "JSON Scalar.lvclass">)  [unwired: 8 in]
                    }
                    n136 = call "Write Array.vi"("error in (no error)"=w472, "Array"=w473) -> ("error out"=w471:errorcluster, "JSON Array out"=w470:refnum<class "JSON Array.lvclass">)  [unwired: 8 in]
                  }
                  n137 = call "Write Array.vi"("error in (no error)"=w463, "Array"=w464) -> ("error out"=w462:errorcluster, "JSON Array out"=w461:refnum<class "JSON Array.lvclass">)  [unwired: 8 in]
                }
                frame "U64" {
                  n138 = Variant To Data(error in=w484, type=u64[][] [], Variant=w487) -> (data=w485:u64[][], error out=w479:errorcluster)
                  n139 = for {
                    tunnel: w485 -> [w493] mode=indexing
                    tunnel: [w489] -> w483 mode=indexing
                    shift-right: [w490] -> w482
                    shift-left: w479 -> [w488]
                    n140 = for {
                      tunnel: w493 -> [w494] mode=indexing
                      shift-right: [w496] -> w491
                      shift-left: w488 -> [w497]
                      tunnel: [w495] -> w492 mode=indexing
                      n141 = call-poly "Set (polymorphic).vi"("error in (no error)"=w497, "Numeric"=w494) -> ("error out"=w496:errorcluster, "JSON Scalar out"=w495:refnum<class "JSON Scalar.lvclass">)  [unwired: 8 in]
                    }
                    n142 = call "Write Array.vi"("error in (no error)"=w491, "Array"=w492) -> ("error out"=w490:errorcluster, "JSON Array out"=w489:refnum<class "JSON Array.lvclass">)  [unwired: 8 in]
                  }
                  n143 = call "Write Array.vi"("error in (no error)"=w482, "Array"=w483) -> ("error out"=w481:errorcluster, "JSON Array out"=w480:refnum<class "JSON Array.lvclass">)  [unwired: 8 in]
                }
              }
            }
            frame 3 {
              n144 = Variant To Data(error in=w504, type=variant[][][] [], Variant=w507) -> (data=w501:variant[][][], error out=w500:errorcluster)
              n145 = for {
                tunnel: w501 -> [w512] mode=indexing
                shift-right: [w510] -> w498
                shift-left: w500 -> [w511]
                tunnel: [w509] -> w499 mode=indexing
                tunnel: w503 -> [w508]
                n146 = call "Variant to JSON.vi"("Treatment of Infinity/NaN"=w508, "error in (no error)"=w511, "Variant"=w512) -> ("error out"=w510:errorcluster, "JSON Value out"=w509:refnum<class "JSON Value.lvclass">)  [unwired: 7 in]
              }
              n147 = call "Write Array.vi"("error in (no error)"=w498, "Array"=w499) -> ("error out"=w506:errorcluster, "JSON Array out"=w505:refnum<class "JSON Array.lvclass">)  [unwired: 8 in]
            }
            frame 4 {
              n148 = Variant To Data(error in=w519, type=variant[][][][] [], Variant=w522) -> (data=w516:variant[][][][], error out=w515:errorcluster)
              n149 = for {
                tunnel: w516 -> [w527] mode=indexing
                shift-right: [w525] -> w513
                shift-left: w515 -> [w526]
                tunnel: [w524] -> w514 mode=indexing
                tunnel: w518 -> [w523]
                n150 = call "Variant to JSON.vi"("Treatment of Infinity/NaN"=w523, "error in (no error)"=w526, "Variant"=w527) -> ("error out"=w525:errorcluster, "JSON Value out"=w524:refnum<class "JSON Value.lvclass">)  [unwired: 7 in]
              }
              n151 = call "Write Array.vi"("error in (no error)"=w513, "Array"=w514) -> ("error out"=w521:errorcluster, "JSON Array out"=w520:refnum<class "JSON Array.lvclass">)  [unwired: 8 in]
            }
            frame 5 {
              n152 = Variant To Data(error in=w534, type=variant[][][][][] [], Variant=w537) -> (data=w531:variant[][][][][], error out=w530:errorcluster)
              n153 = for {
                tunnel: w531 -> [w542] mode=indexing
                shift-right: [w540] -> w528
                shift-left: w530 -> [w541]
                tunnel: [w539] -> w529 mode=indexing
                tunnel: w533 -> [w538]
                n154 = call "Variant to JSON.vi"("Treatment of Infinity/NaN"=w538, "error in (no error)"=w541, "Variant"=w542) -> ("error out"=w540:errorcluster, "JSON Value out"=w539:refnum<class "JSON Value.lvclass">)  [unwired: 7 in]
              }
              n155 = call "Write Array.vi"("error in (no error)"=w528, "Array"=w529) -> ("error out"=w536:errorcluster, "JSON Array out"=w535:refnum<class "JSON Array.lvclass">)  [unwired: 8 in]
            }
            frame Default {
              n156 = Format Into String(format string="Can't support array of dim=%d", w547) -> (resulting string=w544:string)  [unwired: 2 in, 1 out]
              n157 = call <vilib>:"Error Cluster From Error Code.vi"("error in (no error)"=w546, "error message (\"\")"=w544, "error code (0)"=1) -> ("error out"=w549:errorcluster)  [unwired: 6 in]
              n158 = call-poly "Set (polymorphic).vi"() -> ("JSON Scalar out"=w548:refnum<class "JSON Scalar.lvclass">)  [unwired: 10 in, 1 out]
            }
          }
        }
        frame "Cluster" {
          n159 = Variant To Data(error in=w555, type=variant[] [], Variant=w557) -> (data=w551:variant[], error out=w556:errorcluster)
          n160 = Index Array(array=w551) -> (element=w552:variant)  [unwired: 1 in]
          n161 = call <vilib>:"GetTypeInfo.vi"("Variant"=w552) -> ("Name"=w550:string)  [unwired: 6 in, 4 out]
          n162 = case shown="\"\", \"<JSON>\"" w550 {
            tunnel: [w564 w581] -> w559
            tunnel: [w563 w586] -> w558
            tunnel: w556 -> [w562 w585]
            tunnel: w554 -> [w561 w584]
            tunnel: w551 -> [w560 w583]
            frame Default {
              n163 = for {
                shift-right: [w576] -> w564
                shift-left: refnum<class "JSON Object.lvclass"> refnum ("JSON Object out") -> [w575]
                shift-right: [w573] -> w563
                shift-left: w562 -> [w567]
                tunnel: w560 -> [w571] mode=indexing
                tunnel: w561 -> [w570]
                n164 = call <vilib>:"GetTypeInfo.vi"("error in (no error)"=w567, "Variant"=w571) -> ("error out"=w566:errorcluster, "Name"=w568:string, "Type Enum"=w569:T2)  [unwired: 5 in, 2 out]
                n165 = case shown="\"String\"" w569 {
                  tunnel: w568 -> [w578 w580]
                  tunnel: [w578 w579] -> w572
                  frame Default {
                  }
                  frame "String" {
                    n166 = call "Remove JSON Tag.vi"("Name"=w580) -> ("Name (tag stripped)"=w579:string)  [unwired: 9 in, 1 out]
                  }
                }
                n167 = call "Variant to JSON.vi"("Treatment of Infinity/NaN"=w570, "error in (no error)"=w566, "Variant"=w571) -> ("error out"=w574:errorcluster, "JSON Value out"=w577:refnum<class "JSON Value.lvclass">)  [unwired: 7 in]
                n168 = call-dynamic "Set Item by name.vi"("error in (no error)"=w574, "Value"=w577, "name"=w572, "JSON Object in"=w575) -> ("error out"=w573:errorcluster, "JSON Object out"=w576:refnum<class "JSON Object.lvclass">)  [unwired: 5 in, 1 out]
              }
            }
            frame "", "<JSON>" {
              # "Cluster of unnamed (possibly with <JSON>tags) to JSON Array?"
              n169 = for {
                shift-right: [w589] -> w586
                shift-left: w585 -> [w587]
                tunnel: w583 -> [w591] mode=indexing
                tunnel: w584 -> [w590]
                tunnel: [w588] -> w582 mode=indexing
                n170 = call "Variant to JSON.vi"("Treatment of Infinity/NaN"=w590, "error in (no error)"=w587, "Variant"=w591) -> ("error out"=w589:errorcluster, "JSON Value out"=w588:refnum<class "JSON Value.lvclass">)  [unwired: 7 in]
              }
              n171 = call "Write Array.vi"("Array"=w582) -> ("JSON Array out"=w581:refnum<class "JSON Array.lvclass">)  [unwired: 9 in, 1 out]
            }
          }
        }
        frame "Variant", "LV Variant" {
          n172 = Variant To Data(error in=w593, type=variant, Variant=w594) -> (data=w597:variant, error out=w596:errorcluster)
          n173 = call "Variant to JSON.vi"("Treatment of Infinity/NaN"=w592, "error in (no error)"=w596, "Variant"=w597) -> ("error out"=w598:errorcluster, "JSON Value out"=w599:refnum<class "JSON Value.lvclass">)  [unwired: 7 in]
        }
        frame "Waveform" {
          n174 = Variant To Data(error in=w604, type=waveform(dbl) {"t0"=timestamp(0 s since 1904-01-01), "dt"=1.0, "Y"=[]} ("waveform"), Variant=w605) -> (data=w601:waveform(dbl), error out=w600:errorcluster)
          n175 = call "Set Waveform.vi"("Treatment of Infinity/NaN"=w603, "error in (no error)"=w600, "waveform"=w601) -> ("error out"=w606:errorcluster, "JSON Object out"=w607:refnum<class "JSON Object.lvclass">)  [unwired: 7 in]
        }
        frame "Timestamp" {
          n176 = Variant To Data(error in=w608, type=timestamp(0 s since 1904-01-01), Variant=w612) -> (data=w610:timestamp, error out=w609:errorcluster)
          n177 = call-poly "Set (polymorphic).vi"("error in (no error)"=w609, "Time Stamp"=w610) -> ("error out"=w613:errorcluster, "JSON Scalar out"=w614:refnum<class "JSON Scalar.lvclass">)  [unwired: 8 in]
        }
        frame "Refnum" {
          n178 = call <vilib>:"GetRefnumInfo.vi"("error in (no error)"=w617, "Variant"=w618) -> ("error out"=w621:errorcluster, "ReferenceType"=w619:T3)  [unwired: 6 in, 2 out]
          n179 = case shown="\"Visa\", \"IVI\", \"UserDefinedRefnumTag\"" w619 {
            selector: w619 -> [w625 _ _]
            tunnel: [w624 w628 w632] -> w620
            tunnel: w621 -> [w626 w630 w634]
            tunnel: [w623 w627 w633] -> w622
            tunnel: w618 -> [_ w631 w637]
            frame "NotARefnum", "UnknownRefnum" {
              n180 = call <userlib>:"Get Strings from Enum__ogtk.vi"("error in (no error)"=w626, "Enum"=w625) -> ("error out"=w623:errorcluster, "String Value"=w624:string)  [unwired: 6 in, 2 out]
            }
            frame "Visa", "IVI", "UserDefinedRefnumTag" {
              n181 = Variant To Data(error in=w630, type="", Variant=w631) -> (data=w628:string, error out=w627:errorcluster)
            }
            frame Default {
              n182 = Variant To Flattened String(Variant=w637) -> (data string=w636:string)  [unwired: 1 out]
              n183 = Type Cast(type=0, x=w636) -> (*(type *) &x=w635:i32)
              n184 = Format Into String(error in=w634, w635) -> (resulting string=w632:string, error out=w633:errorcluster)  [unwired: 2 in]
            }
          }
          n185 = call-poly "Set (polymorphic).vi"("error in (no error)"=w622, "String"=w620) -> ("error out"=w615:errorcluster, "JSON Scalar out"=w616:refnum<class "JSON Scalar.lvclass">)  [unwired: 8 in]
        }
        frame "LabVIEW Class Instance" {
          w643 = refnum<class "JSON Value.lvclass"> refnum  # JSON Value
          n186 = Variant To Data(error in=w647, type=refnum<class> refnum ("LabVIEW Object"), Variant=w648) -> (data=w644:refnum<class>, error out=w639:errorcluster)
          n187 = To More Specific Class(target class=w643, reference=w644, error in=w639) -> (error out=w645:errorcluster)  [unwired: 1 out]
          n188 = case shown="Pas d'erreur" w645 {
            selector: w645 -> [w649 _]
            tunnel: w644 -> [w653 w658]
            tunnel: w643 -> [w652 _]
            tunnel: [w651 w656] -> w642
            tunnel: [w650 w654] -> w640
            frame No Error {
              # "A JSON Value already, so just\nuse it"
              n189 = To More Specific Class(target class=w652, reference=w653, error in=w649) -> (specific class reference=w651:refnum<class "JSON Value.lvclass">, error out=w650:errorcluster)
            }
            frame Error {
              # "For lack of a better thing to do,\nflatten to string."
              n190 = Flatten To String(anything=w658) -> (data string=w657:string, error out=w655:errorcluster)  [unwired: 3 in, 1 out]
              n191 = call "Set String.vi"("error in (no error)"=w655, "String"=w657) -> ("error out"=w654:errorcluster, "JSON Scalar out"=w656:refnum<class "JSON Scalar.lvclass">)  [unwired: 8 in]
            }
          }
          n192 = Merge Errors(w639, w640) -> (w641:errorcluster)
        }
        frame Default {
          # "For lack of a better thing to do,\nflatten to string."
          n193 = Variant To Flattened String(Variant=w660) -> (data string=w659:string)  [unwired: 1 out]
          n194 = call "Set String.vi"("error in (no error)"=w661, "String"=w659) -> ("error out"=w662:errorcluster, "JSON Scalar out"=w663:refnum<class "JSON Scalar.lvclass">)  [unwired: 8 in]
        }
      }
    }
    frame Error {
    }
  }
  "error out" <- w4
  "JSON Value out" <- w3
